vi "Configure Waveform Characteristics(Amplitude).vi"(0 "VISA resource name":refnum<visa-resource-name>, 1 "High Level (2.5 V)":dbl=2.5, 2 "DC Offset (0 V)":dbl, 5 "Output Channel (1: Channel 1)":i32(ring)=1 items=["Channel 1"=1, "Channel 2"=2], 7 "Amplitude (5)":dbl=5.0, 9 "Amplitude Unit (0: Vpp)":i32(ring) items=["Vpp", "Vrms", "dBm"], 11 "error in (no error)":errorcluster, 12 "Low Level (-2.5 V)":dbl=-2.5) -> (4 "VISA resource name out":refnum<visa-resource-name>, 15 "error out":errorcluster)   [LabVIEW 2012, in "RIGOL DG4000 Series.lvlib"]
doc: "Configures the waveform amplitude settings."
uses:
  <instrlib>/RIGOL DG4000 Series/RIGOL DG4000 Series.lvlib
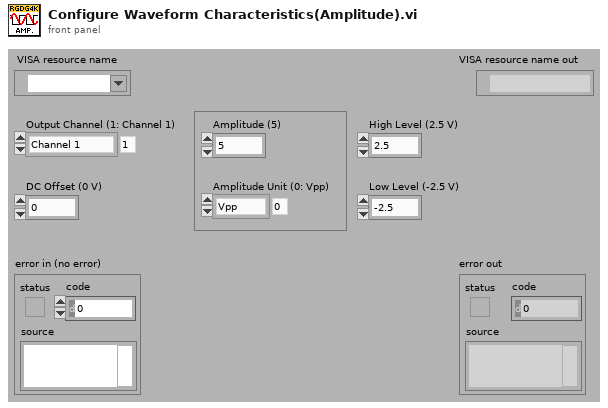
[diagram p1: front panel]
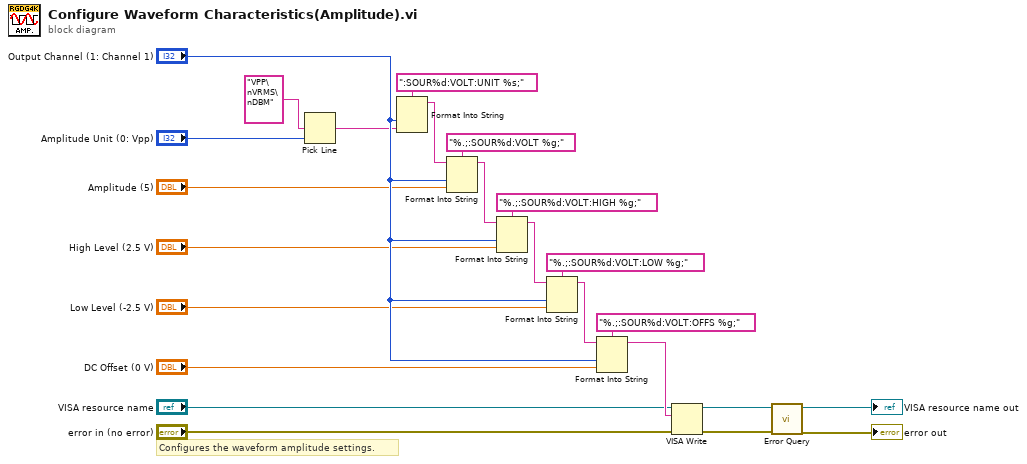
[diagram p0: block diagram]
diagram:
  # "Configures the waveform amplitude settings."
  n1 = Pick Line(multi-line string="VPP\nVRMS\nDBM", line index="Amplitude Unit (0: Vpp)") -> (output string=w20:string)  [unwired: 1 out]
  n2 = Format Into String(format string=":SOUR%d:VOLT:UNIT %s;", "Output Channel (1: Channel 1)", w20) -> (resulting string=w19:string)  [unwired: 2 in, 1 out]
  n3 = Format Into String(format string="%.;:SOUR%d:VOLT %g;", initial string=w19, "Output Channel (1: Channel 1)", "Amplitude (5)") -> (resulting string=w16:string)  [unwired: 1 in, 1 out]
  n4 = Format Into String(format string="%.;:SOUR%d:VOLT:HIGH %g;", initial string=w16, "Output Channel (1: Channel 1)", "High Level (2.5 V)") -> (resulting string=w13:string)  [unwired: 1 in, 1 out]
  n5 = Format Into String(format string="%.;:SOUR%d:VOLT:LOW %g;", initial string=w13, "Output Channel (1: Channel 1)", "Low Level (-2.5 V)") -> (resulting string=w10:string)  [unwired: 1 in, 1 out]
  n6 = Format Into String(format string="%.;:SOUR%d:VOLT:OFFS %g;", initial string=w10, "Output Channel (1: Channel 1)", "DC Offset (0 V)") -> (resulting string=w7:string)  [unwired: 1 in, 1 out]
  n7 = VISA Write(VISA resource name="VISA resource name", write buffer=w7, error in (no error)="error in (no error)") -> (VISA resource name out=w4:refnum<visa-resource-name>, error out=w3:errorcluster)  [unwired: 1 out]
  n8 = call <instrlib>:"Error Query.vi"("error in (no error)"=w3, "VISA resource name"=w4) -> ("error out"=→"error out":errorcluster, "VISA resource name out"=→"VISA resource name out":refnum<visa-resource-name>)  [unwired: 8 out]
